vi "Stepper L298 Drive.vi"(0 "Target Angle (0to90)":dbl, 5 "Start Location Step (0to3)":dbl, 7 "Angle Tolerance (°)":dbl, 9 "stop":bool, 11 "error in (no error)":errorcluster) -> (4 "Current Motor Step (0to3)":dbl, 15 "error out":errorcluster)   [LabVIEW 2017]
uses:
  <vilib>/myRIO/Instrument Drivers/Onboard IO/DIO/typedefs/DIO Reference.ctl
  <vilib>/myRIO/Common/Instrument Driver Framework/Utilities/typedefs/myRIO Generic Hardware Reference.ctl
  <vilib>/myRIO/Common/Instrument Driver Framework/Utilities/typedefs/Hardware Version Enum.ctl
  <vilib>/myRIO/Common/Instrument Driver Framework/Utilities/typedefs/myRIO v1.0 Reference.ctl
  <vilib>/myRIO/Common/Instrument Driver Framework/Utilities/typedefs/Generic FPGA Reference.ctl
  <vilib>/myRIO/Common/Instrument Driver Framework/myRIO v1.0/DIO/typedefs/DIO Channels List.ctl
  <vilib>/myRIO/Common/Instrument Driver Framework/myRIO v1.0/DIO/typedefs/DIO Channels Enum.ctl
  <vilib>/userdefined/High Color/nirio_resource_hc.ctl
  <vilib>/myRIO/Common/Instrument Driver Framework/Utilities/vis/Is FPGA Ref Available.vi
  <vilib>/myRIO/Common/Instrument Driver Framework/myRIO v1.0/DIO/vis/myRIO v1.1 Open DIO.vi
  <vilib>/myRIO/Instrument Drivers/Onboard IO/DIO/vis/Write.vi
  <vilib>/myRIO/Common/Instrument Driver Framework/Utilities/vis/Validate Channels.vi
  <vilib>/myRIO/Common/Instrument Driver Framework/myRIO v1.0/DIO/vis/myRIO v1.0 Reserve DIO.vi
  <vilib>/myRIO/Common/Instrument Driver Framework/myRIO v1.0/Resource Manager/vis/myRIO v1.0 Reserve Channel List.vi
  <vilib>/myRIO/Common/Instrument Driver Framework/myRIO v1.0/DIO/vis/myRIO v1.0 Build MUX Configuration DIO.vi
  <vilib>/myRIO/Common/Instrument Driver Framework/myRIO v1.0/Resource Manager/vis/myRIO v1.0 Reserve Channel.vi
  <vilib>/myRIO/Common/Instrument Driver Framework/myRIO v1.0/Resource Manager/vis/myRIO v1.0 Unreserve Channel.vi
  <vilib>/myRIO/Common/Instrument Driver Framework/myRIO v1.0/Resource Manager/vis/myRIO v1.0 Create Configuration List.vi
  <vilib>/myRIO/Common/Instrument Driver Framework/myRIO v1.0/Resource Manager/vis/myRIO v1.0 Build Mutex Name.vi
  <vilib>/Utility/VariantDataType/GetNumericInfo.vi
  <vilib>/Utility/error.llb/Error Cluster From Error Code.vi
  <vilib>/myRIO/Common/Instrument Driver Framework/myRIO v1.0/myRIO v1.1 Open.vi
  <vilib>/myRIO/Common/Instrument Driver Framework/Utilities/vis/IO Manager.vi
  <vilib>/myRIO/Common/Instrument Driver Framework/Utilities/vis/Configuration Manager.vi
  <vilib>/myRIO/Common/Instrument Driver Framework/myRIO v1.0/Resource Manager/vis/myRIO v1.0 Configure IO.vi
  <vilib>/myRIO/Common/Instrument Driver Framework/myRIO v1.0/myRIO v1.0 Close.vi
  <vilib>/myRIO/Common/Instrument Driver Framework/myRIO v1.0/DIO/vis/myRIO v1.0 Write DIO.vi
  <vilib>/myRIO/Express VI/Onboard IO/DO/DO Express VI.xnode
  <vilib>/myRIO/Instrument Drivers/Onboard IO/DIO/vis/myRIO DIO Open.xnode
  <vilib>/myRIO/Instrument Drivers/Onboard IO/DIO/DIO.lvlib
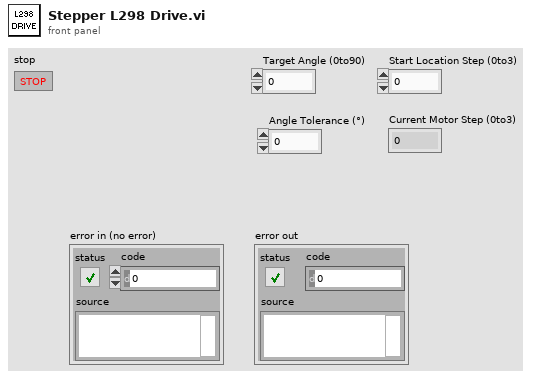
[diagram p1: front panel]
types:
  T1 = typedef "DIO.lvlib/DIO Reference.ctl" = cluster{"myRIO Reference":T2, "DIO Channels List":T6}
  T2 = typedef "myRIO Generic Hardware Reference.ctl" = cluster{"myRIO Model":T3, "myRIO Hardware Reference":T4}
  T3 = typedef "Hardware Version Enum.ctl" = enum16{"Unknown", "myRIO-1900", "myRIO-1950", "roboRIO", "NI ELVIS RIO CM"}
  T4 = typedef "myRIO v1.0 Reference.ctl" = cluster{"Generic FPGA Reference":T5, "Allow multiple opens":bool}
  T5 = typedef "Generic FPGA Reference.ctl" = refnum<k20>
  T6 = typedef "DIO Channels List.ctl" = T7[]
  T7 = typedef "DIO Channels Enum.ctl" = enum16{"Not Connected", "C/DIO0", "C/DIO1", "C/DIO2", "C/DIO3", "C/DIO4", "C/DIO5", "C/DIO6", "C/DIO7", "A/DIO0", "A/DIO1", "A/DIO2", "A/DIO3", "A/DIO4", "A/DIO5", "A/DIO6", "A/DIO7", "A/DIO8", "A/DIO9", "A/DIO10", "A/DIO11", "A/DIO12", "A/DIO13", "A/DIO14", "A/DIO15", "B/DIO0", "B/DIO1", "B/DIO2", "B/DIO3", "B/DIO4", "B/DIO5", "B/DIO6", "B/DIO7", "B/DIO8", "B/DIO9", "B/DIO10", "B/DIO11", "B/DIO12", "B/DIO13", "B/DIO14", "B/DIO15", "LED0", "LED1", "LED2", "LED3", "Button0", "DIO/DIO0", "DIO/DIO1", "DIO/DIO2", "DIO/DIO3", "DIO/DIO4", "DIO/DIO5", "DIO/DIO6", "DIO/DIO7", "DIO/DIO8", "DIO/DIO9", "SPI/CS0", "SPI/CS1", "SPI/CS2", "SPI/CS3", "LED RADIO (Green)", "LED RADIO (Red)", "LED COMM (Green)", "LED COMM (Red)", "LED MODE (Green)", "LED MODE (Red)"}
  T8 = typedef "nirio_resource_hc.ctl" = tag
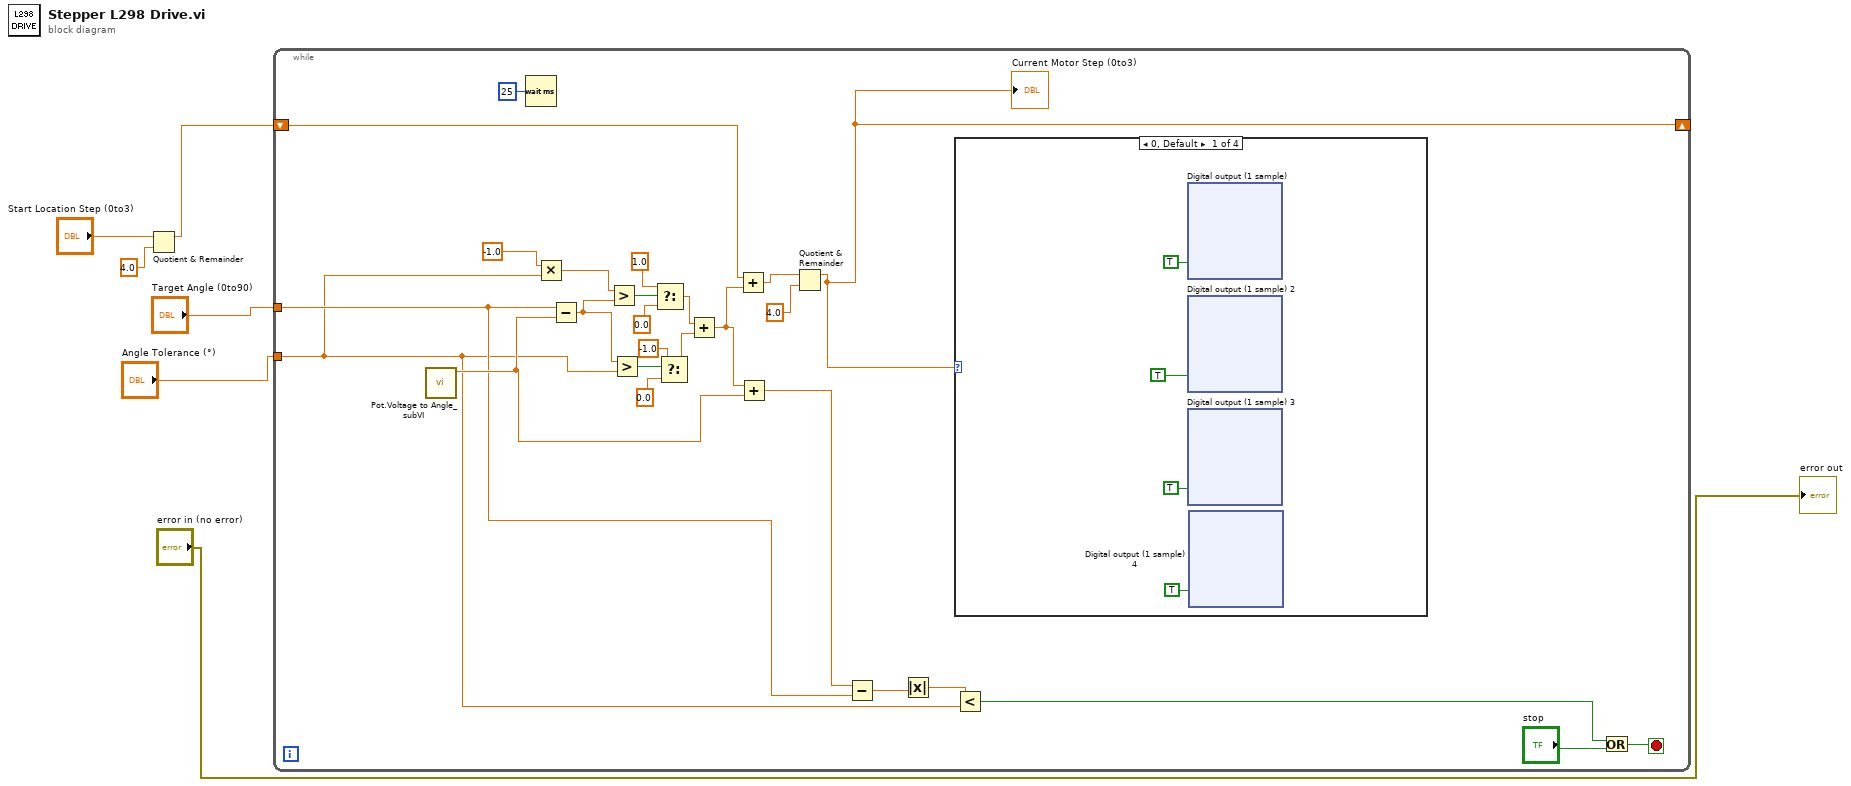
[diagram p0: block diagram]
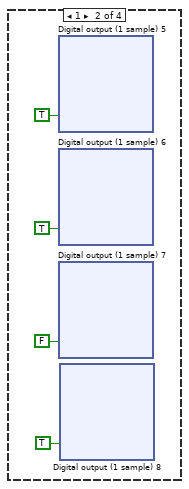
[diagram p2: hidden frame]
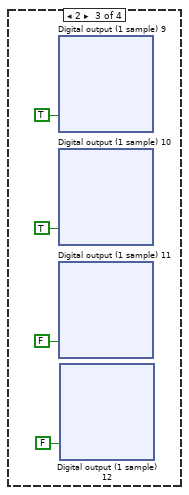
[diagram p3: hidden frame]
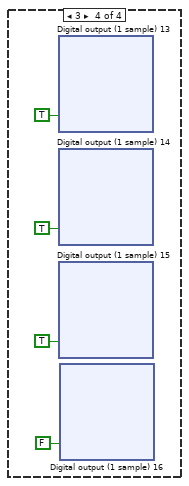
[diagram p4: hidden frame]
diagram:
  n1 = Quotient & Remainder(x="Start Location Step (0to3)", y=4.0) -> (x-y*floor(x/y)=w3:dbl)  [unwired: 1 out]
  n2 = while {
    tunnel: "Target Angle (0to90)" -> [w11]
    shift-right: [w20] -> _
    shift-left: w3 -> [w21]
    tunnel: "Angle Tolerance (°)" -> [w8]
    stop <- w18 stop-if-true
    n3 = call "Pot.Voltage to Angle_subVI.vi"() -> ("Pull-back angle (°)"=w15:dbl)  [unwired: 11 in]
    n4 = Wait (ms)(milliseconds to wait=u32 25) -> ()  [unwired: 1 out]
    n5 = Multiply(x=-1.0, y=w8) -> (x*y=w13:dbl)
    n6 = Subtract(x=w11, y=w15) -> (x-y=w32:dbl)
    n7 = Greater?(x=w13, y=w32) -> (0:w31:bool)
    n8 = Greater?(x=w32, y=w8) -> (0:w28:bool)
    n9 = Select(t=1.0, s=w31, f=0.0) -> (s? t:f=w25:dbl)
    n10 = Select(t=-1.0, s=w28, f=0.0) -> (s? t:f=w24:dbl)
    n11 = Add(x=w25, y=w24) -> (x+y=w19:dbl)
    n12 = Add(x=w21, y=w19) -> (x+y=w23:dbl)
    n13 = Add(x=w19, y=w15) -> (x+y=w12:dbl)
    n14 = Quotient & Remainder(x=w23, y=4.0) -> (x-y*floor(x/y)=w20:dbl)  [unwired: 1 out]
    "Current Motor Step (0to3)" <- w20
    n15 = Subtract(x=w12, y=w11) -> (x-y=w10:dbl)
    n16 = Absolute Value(x=w10) -> (abs(x)=w9:dbl)
    n17 = case shown="0, Default" w20 {
      frame 0, Default {
        n18 = xnode "Digital output (1 sample)"("C/DIO4 (DIO4)"=TRUE) -> ()  [unwired: 1 in, 1 out]
        n19 = xnode "Digital output (1 sample) 2"("A/DIO10 (Pin 31)"=TRUE ("C/DIO2 (DIO2)")) -> ()  [unwired: 1 in, 1 out]
        n20 = xnode "Digital output (1 sample) 3"("C/DIO5 (DIO5)"=TRUE) -> ()  [unwired: 1 in, 1 out]
        n21 = xnode "Digital output (1 sample) 4"("C/DIO3 (DIO3)"=TRUE) -> ()  [unwired: 1 in, 1 out]
      }
      frame 1 {
        n22 = xnode "Digital output (1 sample) 5"("C/DIO4 (DIO4)"=TRUE) -> ()  [unwired: 1 in, 1 out]
        n23 = xnode "Digital output (1 sample) 6"("A/DIO10 (Pin 31)"=TRUE ("C/DIO2 (DIO2)")) -> ()  [unwired: 1 in, 1 out]
        n24 = xnode "Digital output (1 sample) 7"("C/DIO5 (DIO5)"=FALSE) -> ()  [unwired: 1 in, 1 out]
        n25 = xnode "Digital output (1 sample) 8"("C/DIO3 (DIO3)"=TRUE) -> ()  [unwired: 1 in, 1 out]
      }
      frame 2 {
        n26 = xnode "Digital output (1 sample) 9"("C/DIO4 (DIO4)"=TRUE) -> ()  [unwired: 1 in, 1 out]
        n27 = xnode "Digital output (1 sample) 10"("A/DIO10 (Pin 31)"=TRUE ("C/DIO2 (DIO2)")) -> ()  [unwired: 1 in, 1 out]
        n28 = xnode "Digital output (1 sample) 11"("C/DIO5 (DIO5)"=FALSE) -> ()  [unwired: 1 in, 1 out]
        n29 = xnode "Digital output (1 sample) 12"("C/DIO3 (DIO3)"=FALSE) -> ()  [unwired: 1 in, 1 out]
      }
      frame 3 {
        n30 = xnode "Digital output (1 sample) 13"("C/DIO4 (DIO4)"=TRUE) -> ()  [unwired: 1 in, 1 out]
        n31 = xnode "Digital output (1 sample) 14"("A/DIO10 (Pin 31)"=TRUE ("C/DIO2 (DIO2)")) -> ()  [unwired: 1 in, 1 out]
        n32 = xnode "Digital output (1 sample) 15"("C/DIO5 (DIO5)"=TRUE) -> ()  [unwired: 1 in, 1 out]
        n33 = xnode "Digital output (1 sample) 16"("C/DIO3 (DIO3)"=FALSE) -> ()  [unwired: 1 in, 1 out]
      }
    }
    n34 = Less?(x=w9, y=w8) -> (x < y?=w7:bool)
    n35 = Or(x=w7, y="stop") -> (x .or. y?=w18:bool)
  }
  "error out" <- "error in (no error)"
